vi "BRig_arrTrig_Cue2Audio_L.vi"() -> (2 "output_Cue2Audio_L":i32)   [LabVIEW 2014]
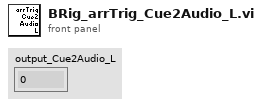
[diagram p1: front panel]
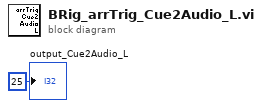
[diagram p0: block diagram]
diagram:
  "output_Cue2Audio_L" <- 25
